vi "Debug - Lower Level - Logging Tool.vi"(8 "Error In":errorcluster, 9 "Data Received":string, 10 "Data Sent":string, 11 "TCP Network Connecion In":refnum<k5>) -> (0 "Error Out":errorcluster, 3 "TCP Network Connecion Out":refnum<k5>)   [LabVIEW 2017, in "Communications Library.lvlib"]
doc: "Adds information to the debug log, every time the error handler is called.\n\nEnable this VI by setting VERBOSE_DEBUG==TRUE, or by setting TCP_DEBUG==TRUE\n(right click on the project in project explorer, select properties, select conditional disable symbols, add VERBOSE_DEBUG and set Value to TRUE)\n\nNote: The error handler is called, regardless of the error state, causing this VI to create a log at the conclussion of every method call at the Mid-Level driver layer."
uses:
  Communications Library.lvlib
  <vilib>/Utility/error.llb/Error Cluster From Error Code.vi
  Typedefs/Debug - TCP Write Type--Enum.ctl
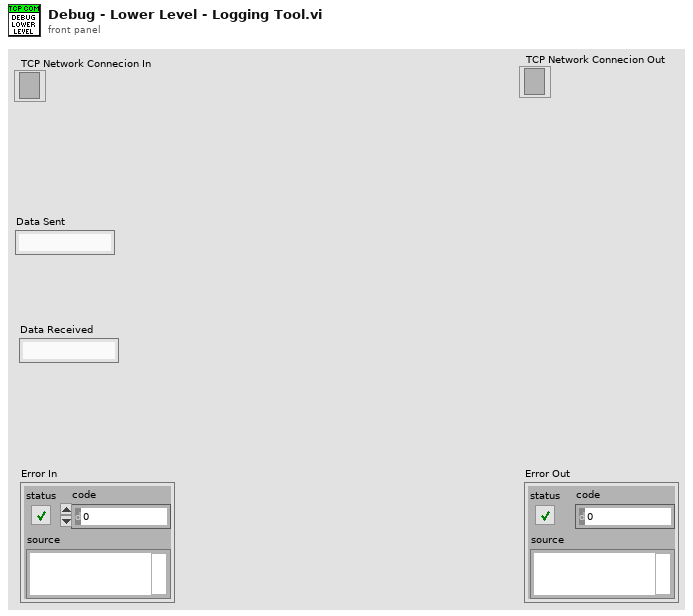
[diagram p1: front panel]
types:
  T1 = typedef "Communications Library.lvlib/Debug - TCP Write Type--Enum.ctl" = enum16{"Log IP and Port Number", "Append New Line"}
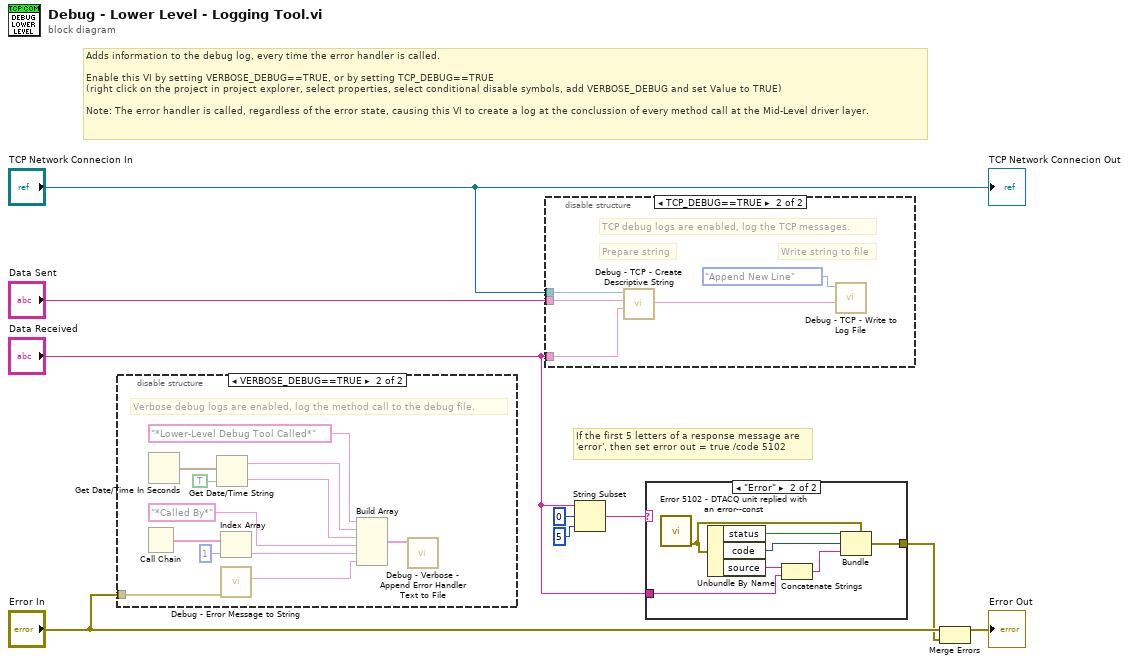
[diagram p0: block diagram]
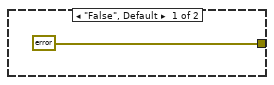
[diagram p2: hidden frame]
diagram:
  # "If the first 5 letters of a response message are\n'error', then set error out = true /code 5102"
  # "Adds information to the debug log, every time the error handler is called.\n\nEnable this VI by setting VERBOSE_DEBUG==TRUE, or by setting TCP_DEBUG==TRUE\n(right click on the project in project explorer, select properties, select conditional disable symbols, add VERBOSE_DEBUG and set Value to TRUE)\n\nNote: The error handler is called, regardless of the error state, causing this VI to create a log at the conclussion of every method call at the Mid-Level driver layer."
  n1 = disable-structure shown="VERBOSE_DEBUG==TRUE" {
    disable-tunnel: "Error In" -> [_ w11]
    frame condition #0 (active) {
    }
    frame condition #1 {
      # "Verbose debug logs are enabled, log the method call to the debug file."
      n2 = Call Chain() -> (call chain=w17:string[])
      n3 = Get Date/Time In Seconds() -> (seconds since 1Jan1904=w16:timestamp)
      n4 = Get Date/Time String(seconds (now)=w16, want seconds? (F)=TRUE) -> (date string=w18:string, time string=w19:string)  [unwired: 1 in]
      n5 = Index Array(array=w17, index=1) -> (element=w20:string)
      n6 = call "Debug - Error Message to String.vi"("error in"=w11) -> ("Error Message"=w10:string)  [unwired: 9 in, 1 out]
      n7 = Build Array("*Lower-Level Debug Tool Called*", w18, w19, "*Called By*", w20, w10) -> (w21:string[])
      n8 = call "Debug - Verbose - Append Error Handler Text to File.vi"("Strings to Append"=w21) -> ()  [unwired: 11 in]
    }
  }
  n9 = disable-structure shown="TCP_DEBUG==TRUE" {
    disable-tunnel: "Data Received" -> [_ w24]
    disable-tunnel: "Data Sent" -> [_ w25]
    disable-tunnel: "TCP Network Connecion In" -> [_ w26]
    frame condition #0 (active) {
    }
    frame condition #1 {
      # "Write string to file"
      # "Prepare string"
      # "TCP debug logs are enabled, log the TCP messages."
      n10 = call "Debug - TCP - Create Descriptive String.vi"("Data Received"=w24, "Data Written"=w25, "TCP Network Connection in"=w26) -> ("Transmission Log"=w22:string)  [unwired: 8 in]
      n11 = call "Debug - TCP - Write to Log File.vi"("Transmission Log (or IP and Port String)"=w22, "Type of Write Opperation"=Debug_-_TCP_Write_Type--Enum."Append New Line") -> ()  [unwired: 10 in]
    }
  }
  n12 = String Subset(string="Data Received", offset (0)=0, length (rest)=5 ("length (rest)")) -> (substring=w3:string)
  n13 = case shown="\"Error\"" w3 {
    tunnel: [errorcluster {"status"=FALSE, "code"=0, "source"=""} ("error constant") w31] -> w2
    tunnel: "Data Received" -> [_ w33]
    frame "False", Default {
    }
    frame "Error" {
      n14 = call "Error 5102 - DTACQ unit replied with an error--const.vi"() -> ("error out"=w32:errorcluster)  [unwired: 11 in]
      n15 = Unbundle By Name(w32) -> ("status"=w29:bool, "code"=w28:i32, "source"=w34:string)
      n16 = Concatenate Strings(w34, w33) -> (w30:string)
      n17 = Bundle(cluster=w32, "status"=w29, "code"=w28, "source"=w30) -> (w31:errorcluster)
    }
  }
  n18 = Merge Errors("Error In", w2) -> (→"Error Out":errorcluster)
  "TCP Network Connecion Out" <- "TCP Network Connecion In"
